vi "SigSyn (G3)-Check Filter Used.vi"(1 "Waveform in":T1) -> (0 "Use filter":bool)   [LabVIEW 2020]
uses:
  XControls/Waveform XControls/Waveform (G3)/Waveform Data.ctl
  Waveform VIs/Waveform Enum (V3).ctl
  XControls/Waveform XControls/Tone (G3)/Tone.Properties.ctl
  Waveform VIs/Pulse Train VIs/Pulse Train Params.ctl
  Waveform VIs/Pulse Train VIs/Pulse Polarity.ctl
  Waveform VIs/Pulse Train VIs/PT-Continuous State.ctl
  Waveform VIs/Noise VIs/Noise (G3).ctl
  Waveform VIs/Noise VIs/Noise (G3).Properties.ctl
  Waveform VIs/Noise VIs/Noise (G3).Data.ctl
  Waveform VIs/File VIs/StimFile-Params.ctl
  Waveform VIs/FM Sweep VIs/FM Sweep Params.ctl
  Waveform VIs/Chirp Train VIs/Chirp Train.ctl
  Waveform VIs/Chirp Train VIs/Chirp Train Params.ctl
  Waveform VIs/Complex Tone VIs/CT-Params.ctl
  Waveform VIs/Complex Tone VIs/CT-Phase Enum.ctl
  Waveform VIs/Complex Tone VIs/CT-Runtime Data.ctl
  XControls/Waveform XControls/FM Tone/Data.ctl
  XControls/Waveform XControls/Vowel/Vowel.Properties.ctl
  Waveform VIs/Ramp VIs/Ramp.Properties.ctl
  XControls/Waveform XControls/Tone (G3)/Tone (G3).xctl
  XControls/Waveform XControls/FM Tone/FM Tone.xctl
  XControls/Waveform XControls/Vowel/Vowel.xctl
  XControls/Waveform XControls/Waveform (G3)/Waveform (G3).xctl
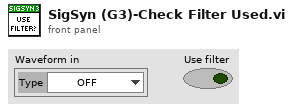
[diagram p1: front panel]
types:
  T1 = typedef "Waveform (G3).xctl/Waveform Data.ctl" = cluster{"Type":T2, "Tone":T3, "Pulse Train":T4, "Noise":T7, "File":T10, "FMSweep":T11, "Chirp Train":T12, "Complex Tone":cluster{"Params":T14, "Data":T16}, "FM":T17, "Vowel":T18, "Ramp":T19}
  T2 = typedef "Waveform Enum (V3).ctl" = enum16{"OFF", "Tone", "Noise", "Pulse Train", "File", "FM Sweep", "Chirp Train", "Complex Tone", "FM Tone", "Vowel", "Ramp"}
  T3 = typedef "Tone (G3).xctl/Tone.Properties.ctl" = cluster{"Frequency (kHz)":dbl, "Phase (cycles)":dbl, "Random phase":bool}
  T4 = typedef "Pulse Train Params.ctl" = cluster{"Pulse width (us)":dbl, "Pulse rate (Hz)":dbl, "Gap (ms)":dbl, "Polarity":T5, "PT State":T6, "Asynch":bool}
  T5 = typedef "Pulse Polarity.ctl" = enum16{"POS", "NEG", "POS-NEG", "NEG-POS"}
  T6 = typedef "PT-Continuous State.ctl" = cluster{"Template":dbl[], "Nperiod":i32, "Index":i32, "Pulse Rate (Hz)":dbl, "Phase (cycles)":dbl, "Noff":i32}
  T7 = typedef "Noise (G3).ctl" = cluster{"Properties":T8, "Data":T9}
  T8 = typedef "Noise (G3).Properties.ctl" = cluster{"InvFilt":bool, "Aweight":bool, "Seed":i32, "Tokens":i32, "Brickwall":bool}
  T9 = typedef "Noise (G3).Data.ctl" = cluster{"TokenNum":i32}
  T10 = typedef "StimFile-Params.ctl" = cluster{"Filename":path, "Signal":dbl[], "Channel":i32, "stream":bool, "offset":i32, "nreps":i32, "loops":i32, "Randomize":bool, "order":i32[], "Seed":i32, "Tokens":i32}
  T11 = typedef "FM Sweep Params.ctl" = cluster{"Rate (oct/s)":dbl, "Fmin (Hz)":dbl, "Fmax (Hz)":dbl, "Ramp (ms)":dbl, "Linear":bool}
  T12 = typedef "Chirp Train.ctl" = cluster{"Params":T13, "Data":cluster{"WF":dbl[]}}
  T13 = typedef "Chirp Train Params.ctl" = cluster{"Fmin (kHz)":dbl, "Fmax (kHz)":dbl, "Compensate":bool, "Duration (ms)":dbl}
  T14 = typedef "CT-Params.ctl" = cluster{"F0 (Hz)":dbl, "Band":cluster{"Flow (Hz)":dbl, "Fhigh (Hz)":dbl}, "Phase":T15, "Min F0 (Hz)":dbl, "Max F0 (Hz)":dbl, "ContinRandPhase":bool, "Max peak factor":dbl, "Max mod depth":dbl, "MinHarmNum":i32, "MaxHarmNum":i32, "Level Mode":enum16{"per component", "overall rms"}, "% jitter":dbl}
  T15 = typedef "CT-Phase Enum.ctl" = enum16{"Cosine", "Random", "Alternating"}
  T16 = typedef "CT-Runtime Data.ctl" = cluster{"Ncomp":i32, "MinHarm":i32, "Phase":dbl[], "Amplitude":dbl[], "Npts/frame":i32, "Last F0":dbl, "Fmin":dbl, "Fmax":dbl, "Lslope":dbl, "randphase":bool, "overall rms":bool, "fmult":dbl[], "jittered":bool}
  T17 = typedef "FM Tone.xctl/Data.ctl" = cluster{"Carrier (kHz)":dbl, "ModRate (Hz)":dbl, "Depth (Hz)":dbl, "Phase (cycles)":dbl}
  T18 = typedef "Vowel.xctl/Vowel.Properties.ctl" = cluster{"Freqs":string, "Set level":enum16{"Total", "Per component"}, "Freq":dbl[], "weights":dbl[]}
  T19 = typedef "Ramp.Properties.ctl" = cluster{"Duration (ms)":dbl}
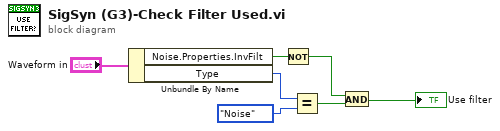
[diagram p0: block diagram]
diagram:
  n1 = Unbundle By Name("Waveform in") -> ("Noise.Properties.InvFilt"=w2:bool, "Type"=w4:T2)
  n2 = Not(x=w2) -> (.not. x?=w1:bool)
  n3 = Equal?(x=w4, y=Waveform_Enum_(V3)."Noise") -> (x = y?=w6:bool)
  n4 = And(x=w1, y=w6) -> (x .and. y?=→"Use filter":bool)
